vi "SHsU(T)-15-07-17.vi"(6 "TemperaturenSH[V]":dbl[](array[numeric]), 9 "Traps/MachKoeff2":dbl[](array[numeric]), 10 "Traps/MachKoeff1":dbl[](array[numeric]), 11 "Traps/MachKoeff0":dbl[](array[numeric])) -> (2 "SpannungenSH":T1 {"setpoint" format="%.23g"; "setpoint" format="%.23g"; "[2]" format="%.23g"; "[3]" format="%.23g"; "[4]" format="%.23g"; "[5]" format="%.23g"})   [LabVIEW 2010]
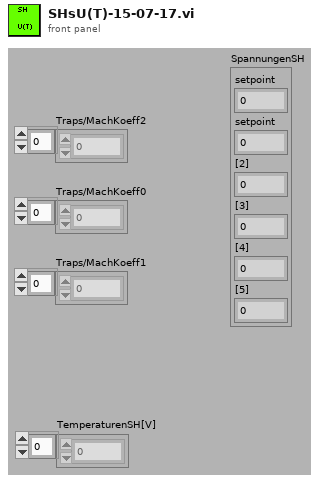
[diagram p1: front panel]
types:
  T1 = cluster{"setpoint":fxp<+/-,26,5>, "setpoint":fxp<+/-,26,5>, "[2]":fxp<+/-,26,5>, "[3]":fxp<+/-,26,5>, "[4]":fxp<+/-,26,5>, "[5]":fxp<+/-,26,5>}
  T2 = cluster{"[0]":fxp<+/-,26,5>, "[1]":fxp<+/-,26,5>, "[2]":fxp<+/-,26,5>, "[3]":fxp<+/-,26,5>, "[4]":fxp<+/-,26,5>, "[5]":fxp<+/-,26,5>}
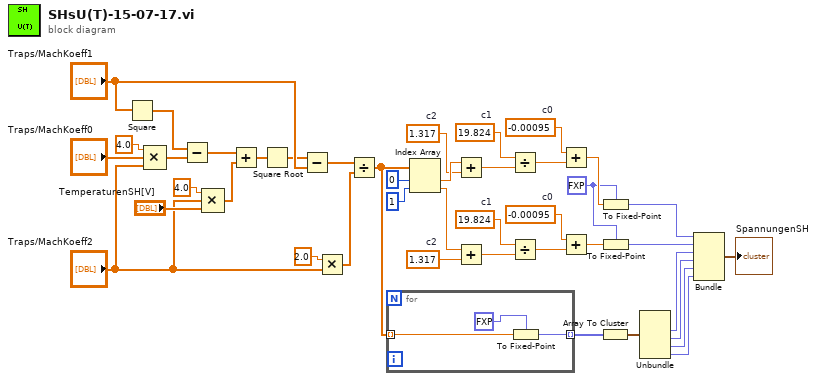
[diagram p0: block diagram]
diagram:
  w3 = fxp<+/-,26,5> 0.0 ("setpoint")
  w8 = -0.00095  # c0
  w10 = 19.824  # c1
  w11 = 1.317  # c2
  w15 = -0.00095  # c0
  w17 = 19.824  # c1
  w18 = 1.317  # c2
  n1 = Square(x="Traps/MachKoeff1") -> (x^2=w38:dbl[])
  n2 = Compound Arithmetic op=MULTIPLY(4.0, "Traps/MachKoeff0", "Traps/MachKoeff2") -> (w37:dbl[])
  n3 = Subtract(x=w38, y=w37) -> (x-y=w36:dbl[])
  n4 = Compound Arithmetic op=MULTIPLY(4.0, "Traps/MachKoeff2", "TemperaturenSH[V]") -> (w35:dbl[])
  n5 = Add(x=w36, y=w35) -> (x+y=w34:dbl[])
  n6 = Square Root(x=w34) -> (sqrt(x)=w1:dbl[])
  n7 = Subtract(x=w1, y="Traps/MachKoeff1") -> (x-y=w32:dbl[])
  n8 = Multiply(x=2.0, y="Traps/MachKoeff2") -> (x*y=w29:dbl[])
  n9 = Divide(x=w32, y=w29) -> (x/y=w27:dbl[])
  n10 = for {
    tunnel: w27 -> [w45] mode=indexing
    tunnel: [w44] -> w26 mode=indexing
    n11 = To Fixed-Point(fixed-point type=fxp<+/-,26,5> 0.0 ("setpoint"), number=w45) -> (fixed-point=w44:fxp<+/-,26,5>)
  }
  n12 = Index Array(array=w27, index #1=0 ("index"), index #2=1 ("index")) -> (element #1=w19:dbl, element #2=w5:dbl)
  n13 = Add(x=w19, y=w18) -> (x+y=w16:dbl)
  n14 = Add(x=w5, y=w11) -> (x+y=w9:dbl)
  n15 = Divide(x=w17, y=w16) -> (x/y=w14:dbl)
  n16 = Divide(x=w10, y=w9) -> (x/y=w7:dbl)
  n17 = Add(x=w15, y=w14) -> (x+y=w13:dbl)
  n18 = Add(x=w8, y=w7) -> (x+y=w6:dbl)
  n19 = Array To Cluster(array=w26) -> (cluster=w25:T2)
  n20 = To Fixed-Point(fixed-point type=w3, number=w13) -> (fixed-point=w12:fxp<+/-,26,5>)
  n21 = To Fixed-Point(fixed-point type=w3, number=w6) -> (fixed-point=w4:fxp<+/-,26,5>)
  n22 = Unbundle(w25) -> ("[2]"=w24:fxp<+/-,26,5>, "[3]"=w23:fxp<+/-,26,5>, "[4]"=w22:fxp<+/-,26,5>, "[5]"=w21:fxp<+/-,26,5>)  [unwired: 2 out]
  n23 = Bundle("setpoint"=w12, "setpoint"=w4, "[2]"=w24, "[3]"=w23, "[4]"=w22, "[5]"=w21) -> (→"SpannungenSH":T1)  [unwired: 1 in]
